vi "Set current pretomo stack.vi"(8 "error in (no error)":errorcluster, 9 "current y stack":i32, 10 "current x stack":i32, 11 "Tomo in":refnum<class "Tomo.lvclass">) -> (0 "error out":errorcluster, 3 "Tomo out":refnum<class "Tomo.lvclass">)   [LabVIEW 2012, in "Tomo.lvclass"]
uses:
  Tomo.lvclass
  Tomo.lvclass/Tomo.ctl
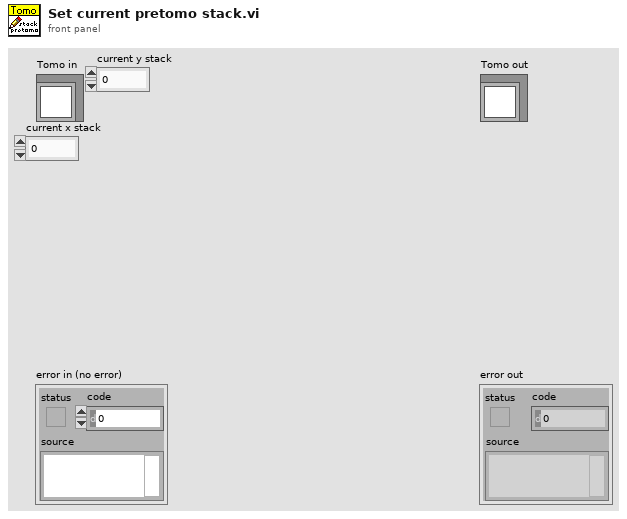
[diagram p1: front panel]
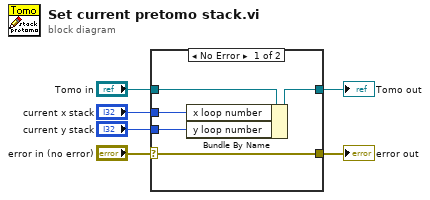
[diagram p0: block diagram]
diagram:
  n1 = case shown="No Error" "error in (no error)" {
    selector: "error in (no error)" -> [w11 w13]
    tunnel: [w11 w13] -> w5
    tunnel: [w9 w12] -> w3
    tunnel: "Tomo in" -> [w10 w12]
    tunnel: "current x stack" -> [w8 _]
    tunnel: "current y stack" -> [w7 _]
    frame No Error {
      n2 = Bundle By Name(cluster=w10, "x loop number"=w8, "y loop number"=w7) -> (w9:refnum<class "Tomo.lvclass">)
    }
    frame Error {
    }
  }
  "error out" <- w5
  "Tomo out" <- w3
